vi "Read Custom VI Mode.vi"(8 "error in (no error)":errorcluster, 11 "Template in":refnum<class "MetaDataObj.lvclass">) -> (0 "error out":errorcluster, 2 "Custom VI Mode":T1, 3 "Template out":refnum<class "MetaDataObj.lvclass">)   [LabVIEW 2016, in "MetaDataObj.lvclass"]
uses:
  <resource>/dialog/NewProjectWizard/MetaDataObj/MetaDataObj.lvclass
  <resource>/dialog/NewProjectWizard/MetaDataObj/Accessors/CustomVIModes.ctl
  <resource>/dialog/NewProjectWizard/MetaDataObj/MetaDataObj.lvclass/MetaDataObj.ctl
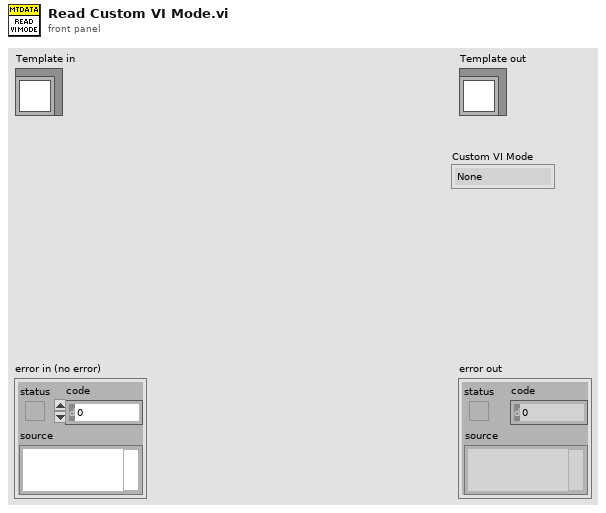
[diagram p1: front panel]
types:
  T1 = typedef "CustomVIModes.ctl" = enum16{"None", "AfterPage1", "AfterPage2WithUI", "AfterPage2NoUI"}
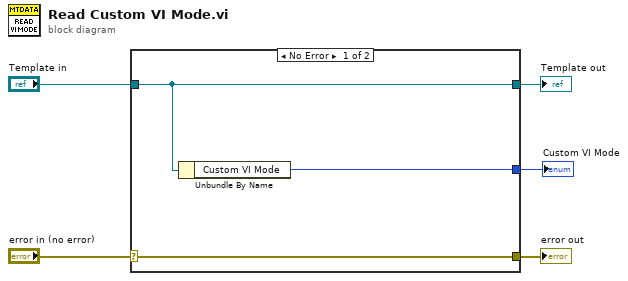
[diagram p0: block diagram]
diagram:
  n1 = case shown="No Error" "error in (no error)" {
    selector: "error in (no error)" -> [w8 w9]
    tunnel: [w8 w9] -> w4
    tunnel: [w7 w10] -> w2
    tunnel: "Template in" -> [w7 w10]
    tunnel: [w6 _] -> w1
    frame No Error {
      n2 = Unbundle By Name(w7) -> ("Custom VI Mode"=w6:T1)
    }
    frame Error {
    }
  }
  "error out" <- w4
  "Template out" <- w2
  "Custom VI Mode" <- w1
